vi "KepcoDCPwr Software Timed current Ramp.vi"(0 "VISA resource name":refnum<visa-resource-name>, 1 "Disable @ End":bool, 2 "Repeat":bool, 3 "# of Cycles":i32, 4 "Model In":string, 5 "Start (current)":dbl format="%.2f", 7 "End (current)":dbl format="%.2f", 8 "OPpen/Close":bool=TRUE, 9 "current Increment":dbl format="%.6f", 11 "error in (no error)":errorcluster, 12 "Dwell (ms)":u32, 13 "Readback Voltage":bool, 14 "Readback Current":bool) -> (6 "actual current":dbl, 15 "error out":errorcluster)   [LabVIEW 2013]
doc: "Current ramp. Execute current steps"
panel:
  out "Cycle Number":i32=1
  in  "Stop Ramp":bool
  out "DC AMPERES":dbl format="%.3f"
  out "DC VOLTS":dbl format="%.3f"
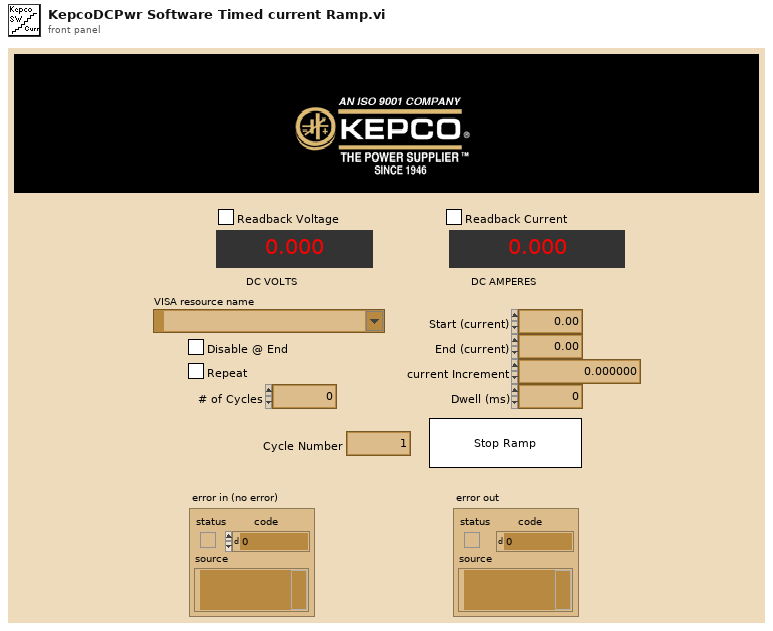
[diagram p1: front panel]
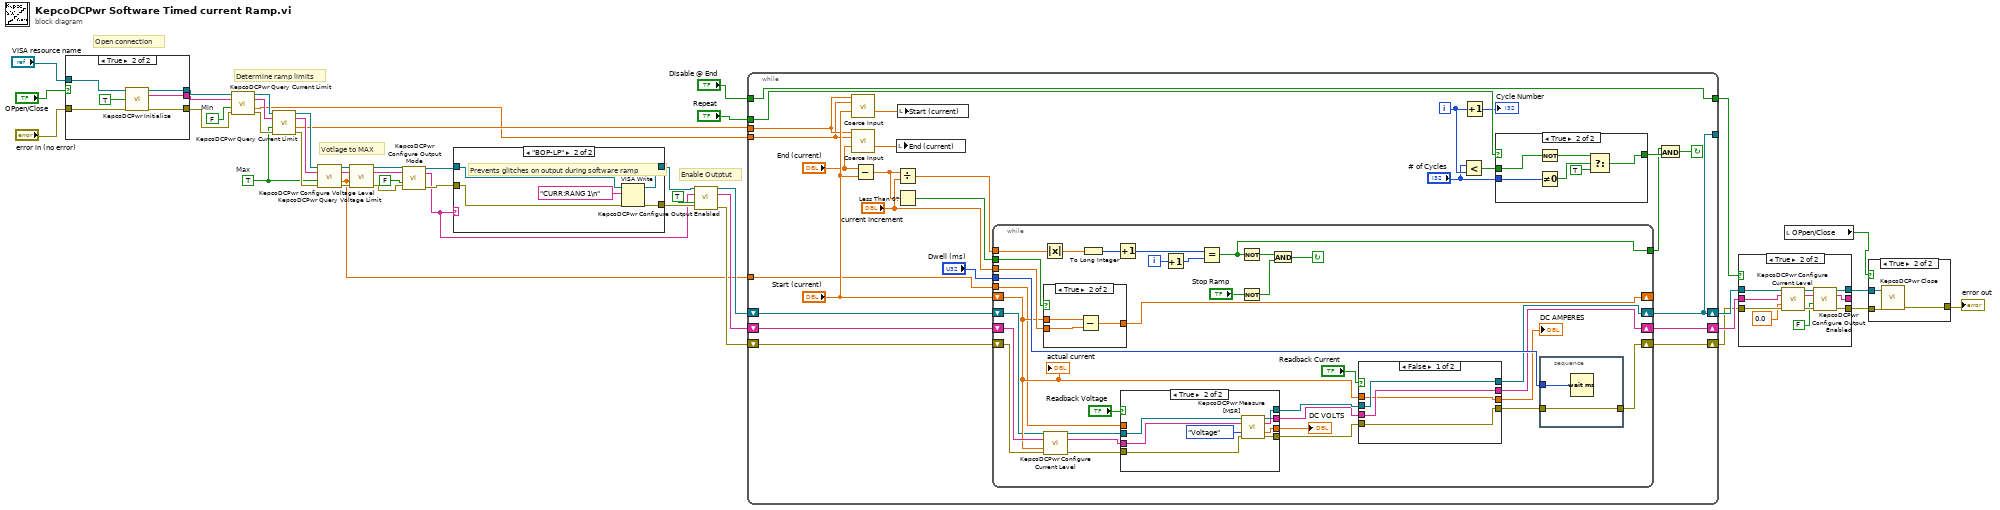
[diagram p0: block diagram]
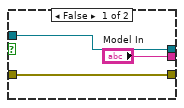
[diagram p3: hidden frame]
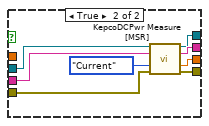
[diagram p5: hidden frame]
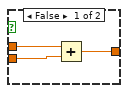
[diagram p7: hidden frame]
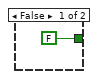
[diagram p8: hidden frame]
diagram:
  w19 = TRUE  # Max
  w24 = FALSE  # Min
  # "Enable Outptut"
  # "Open connection"
  # "Determine ramp limits"
  # "Votlage to MAX"
  n1 = case shown="True" "OPpen/Close" {
    tunnel: "error in (no error)" -> [w45 w51]
    tunnel: [w46 w50] -> w30
    tunnel: ["Model In" w49] -> w27
    tunnel: [w45 w48] -> w26
    tunnel: "VISA resource name" -> [w46 w47]
    frame False {
    }
    frame True {
      n2 = call "KepcoDCPwr Initialize.vi"("VISA Resource Name"=w47, "id query (True)"=TRUE, "error in (no error)"=w51) -> ("VISA Session Out"=w50:refnum<visa-resource-name>, "Model Out"=w49:string, "error out"=w48:errorcluster)  [unwired: 3 in, 7 out]
    }
  }
  n3 = call "KepcoDCPwr Query Current Limit.vi"("VISA Session"=w30, "Model In"=w27, "Level"=w24, "error in (no error)"=w26) -> ("VISA Session Out"=w29:refnum<visa-resource-name>, "Model Out"=w28:string, "current limit"=w13:dbl, "error out"=w25:errorcluster)  [unwired: 1 in, 7 out]
  n4 = call "KepcoDCPwr Query Current Limit.vi"("VISA Session"=w29, "Model In"=w28, "Level"=w19, "error in (no error)"=w25) -> ("VISA Session Out"=w20:refnum<visa-resource-name>, "Model Out"=w21:string, "current limit"=w14:dbl, "error out"=w22:errorcluster)  [unwired: 1 in, 7 out]
  n5 = call "KepcoDCPwr Query Voltage Limit.vi"("VISA Session"=w20, "Model In"=w21, "Max Level (T),MIN LEVEL(F)"=w19, "error in (no error)"=w22) -> ("VISA Session Out"=w16:refnum<visa-resource-name>, "Model Out"=w17:string, "voltage level"=w12:dbl, "error out"=w18:errorcluster)  [unwired: 1 in, 7 out]
  n6 = call "KepcoDCPwr Configure Voltage Level.vi"("VISA Session"=w16, "Model In"=w17, "level (0.0 volts)"=w12, "error in (no error)"=w18) -> ("VISA Session Out"=w7:refnum<visa-resource-name>, "Model Out"=w6:string, "error out"=w5:errorcluster)  [unwired: 1 in, 8 out]
  n7 = call "KepcoDCPwr Configure Output Mode.vi"("VISA Session"=w7, "Model In"=w6, "Mode In (Volt)"=FALSE, "error in (no error)"=w5) -> ("VISA Session Out"=w2:refnum<visa-resource-name>, "Model Out"=w3:string, "error out"=w4:errorcluster)  [unwired: 9 in]
  n8 = case shown="\"BOP-LP\"" w3 {
    tunnel: w4 -> [w54 w59]
    tunnel: [w54 w56] -> w10
    tunnel: [w53 w57] -> w11
    tunnel: w2 -> [w53 w58]
    frame "", "STANDARD", Default {
    }
    frame "BOP-LP" {
      # "Prevents glitches on output during software ramp"
      n9 = VISA Write(VISA resource name=w58, write buffer="CURR:RANG 1\n", error in (no error)=w59) -> (VISA resource name out=w57:refnum<visa-resource-name>, error out=w56:errorcluster)  [unwired: 1 out]
    }
  }
  n10 = call "KepcoDCPwr Configure Output Enabled.vi"("VISA Session"=w11, "Model In"=w3, "Input enabled (True)"=TRUE, "error in (no error)"=w10) -> ("VISA Session Out"=w23:refnum<visa-resource-name>, "Model Out"=w34:string, "error out"=w33:errorcluster)  [unwired: 9 out]
  n11 = while {
    tunnel: [w83] -> _
    shift-left: w23 -> [w63]
    tunnel: w13 -> [w65]
    tunnel: w14 -> [w66]
    tunnel: [w80] -> w36
    tunnel: "Disable @ End" -> [w80]
    tunnel: "Repeat" -> [w86]
    shift-left: w34 -> [w79]
    shift-right: [w82] -> w40
    shift-left: w33 -> [w78]
    shift-right: [w81] -> w39
    shift-right: [w83] -> w41
    tunnel: w12 -> [w60]
    i -> [w62]
    stop <- w71 continue-if-true
    n12 = call "Coerce Input.vi"("Max"=w66, "Min"=w65, "Input"="Start (current)") -> ("Output"=w68:dbl)  [unwired: 12 out]
    n13 = call "Coerce Input.vi"("Max"=w66, "Min"=w65, "Input"="End (current)") -> ("Output"=w64:dbl)  [unwired: 12 out]
    n14 = Subtract(x="End (current)", y="Start (current)") -> (x-y=w75:dbl)
    n15 = Divide(x=w75, y="current Increment") -> (x/y=w73:dbl)
    n16 = local write "End (current)"(w64) -> ()
    n17 = Less Than 0?(x=w75) -> (x < 0?=w74:bool)
    n18 = local write "Start (current)"(w68) -> ()
    n19 = while {
      shift-left: w63 -> [w91]
      tunnel: [w88] -> w70
      tunnel: w73 -> [w113]
      tunnel: w74 -> [w116]
      tunnel: "current Increment" -> [w118]
      shift-left: "Start (current)" -> [w93]
      shift-right: [w117] -> _
      tunnel: "Dwell (ms)" -> [w119]
      shift-left: w79 -> [w95]
      shift-right: [w107] -> w82
      shift-right: [w92] -> w83
      shift-left: w78 -> [w94]
      shift-right: [w120] -> w81
      tunnel: w60 -> [w87]
      i -> [w104]
      stop <- w102 continue-if-true
      n20 = Absolute Value(x=w113) -> (abs(x)=w114:dbl)
      n21 = case shown="True" w116 {
        tunnel: w93 -> [w146 w150]
        tunnel: w118 -> [w145 w149]
        tunnel: [w147 w148] -> w117
        frame False {
          n22 = Add(x=w146, y=w145) -> (x+y=w147:dbl)
        }
        frame True {
          n23 = Subtract(x=w150, y=w149) -> (x-y=w148:dbl)
        }
      }
      n24 = call "KepcoDCPwr Configure Current Level.vi"("VISA Session"=w91, "Model In"=w95, "level (0.0 volts)"=w93, "error in (no error)"=w94) -> ("VISA Session Out"=w96:refnum<visa-resource-name>, "Model Out"=w97:string, "error out"=w98:errorcluster)  [unwired: 1 in, 8 out]
      n25 = To Long Integer(number=w114) -> (32bit integer=w115:i32)
      n26 = Increment(x=w115) -> (x+1=w105:i32)
      n27 = case shown="True" "Readback Voltage" {
        tunnel: [w133 w138] -> w112
        tunnel: w96 -> [w136 w140]
        tunnel: w97 -> [w135 w142]
        tunnel: w98 -> [w134 w144]
        tunnel: [w136 w139] -> w111
        tunnel: [w135 w141] -> w110
        tunnel: [w134 w143] -> w109
        tunnel: w87 -> [w133 _]
        frame False {
        }
        frame True {
          n28 = call "KepcoDCPwr Measure [MSR].vi"("VISA Session"=w140, "Model In"=w142, "measurement type (voltage)"=enum16{"Voltage", "Current"}."Voltage", "error in (no error)"=w144) -> ("VISA Session Out"=w139:refnum<visa-resource-name>, "Model Out"=w141:string, "measurement"=w138:dbl, "error out"=w143:errorcluster)  [unwired: 4 in, 4 out]
        }
      }
      "DC VOLTS" <- w112
      n29 = Increment(x=w104) -> (x+1=w103:i32)
      n30 = Equal?(x=w105, y=w103) -> (x = y?=w88:bool)
      n31 = Not(x=w88) -> (.not. x?=w89:bool)
      n32 = Not(x="Stop Ramp") -> (.not. x?=w90:bool)
      n33 = And(x=w89, y=w90) -> (x .and. y?=w102:bool)
      n34 = case shown="False" "Readback Current" {
        tunnel: [w121 w126] -> w106
        tunnel: w111 -> [w124 w128]
        tunnel: w110 -> [w123 w130]
        tunnel: w109 -> [w122 w132]
        tunnel: [w124 w127] -> w92
        tunnel: [w123 w129] -> w107
        tunnel: [w122 w131] -> w108
        tunnel: w93 -> [w121 _]
        frame False {
        }
        frame True {
          n35 = call "KepcoDCPwr Measure [MSR].vi"("VISA Session"=w128, "Model In"=w130, "measurement type (voltage)"=enum16{"Voltage", "Current"}."Current", "error in (no error)"=w132) -> ("VISA Session Out"=w127:refnum<visa-resource-name>, "Model Out"=w129:string, "measurement"=w126:dbl, "error out"=w131:errorcluster)  [unwired: 4 in, 4 out]
        }
      }
      "DC AMPERES" <- w106
      n36 = stacked-sequence {
        tunnel: w108 -> [w152]
        tunnel: [w152] -> w120
        tunnel: w119 -> [w151]
        frame #0 {
          n37 = Wait (ms)(milliseconds to wait=w151) -> ()  [unwired: 1 out]
        }
      }
      "actual current" <- w93
    }
    n38 = Less?(x="# of Cycles", y=w62) -> (x < y?=w85:bool)
    n39 = Increment(x=w62) -> (x+1=→"Cycle Number":i32)
    n40 = case shown="True" w86 {
      tunnel: [FALSE w155] -> w72
      tunnel: w85 -> [_ w159]
      tunnel: "# of Cycles" -> [_ w158]
      frame False {
      }
      frame True {
        n41 = Not(x=w159) -> (.not. x?=w156:bool)
        n42 = Not Equal To 0?(x=w158) -> (x != 0?=w157:bool)
        n43 = Select(t=w156, s=w157, f=TRUE) -> (s? t:f=w155:bool)
      }
    }
    n44 = And(x=w70, y=w72) -> (x .and. y?=w71:bool)
  }
  n45 = case shown="True" w36 {
    tunnel: w41 -> [w162 w173]
    tunnel: w40 -> [w161 w172]
    tunnel: w39 -> [w160 w171]
    tunnel: [w160 w166] -> w37
    tunnel: [w162 w165] -> w38
    tunnel: [w161 w164] -> _
    frame False {
    }
    frame True {
      n46 = call "KepcoDCPwr Configure Current Level.vi"("VISA Session"=w173, "Model In"=w172, "level (0.0 volts)"=0.0, "error in (no error)"=w171) -> ("VISA Session Out"=w169:refnum<visa-resource-name>, "Model Out"=w168:string, "error out"=w167:errorcluster)  [unwired: 8 in, 1 out]
      n47 = call "KepcoDCPwr Configure Output Enabled.vi"("VISA Session"=w169, "Model In"=w168, "Input enabled (True)"=FALSE ("output enabled (True)"), "error in (no error)"=w167) -> ("VISA Session Out"=w165:refnum<visa-resource-name>, "Model Out"=w164:string, "error out"=w166:errorcluster)  [unwired: 9 out]
    }
  }
  n48 = local read "OPpen/Close"() -> (w8:bool)
  n49 = case shown="True" w8 {
    tunnel: w38 -> [_ w177]
    tunnel: w37 -> [w174 w176]
    tunnel: [w174 w175] -> w32
    frame False {
    }
    frame True {
      n50 = call "KepcoDCPwr Close.vi"("VISA Session"=w177, "error in (no error)"=w176) -> ("error out"=w175:errorcluster)  [unwired: 13 out]
    }
  }
  "error out" <- w32
